vi "DVR unwrapper.vi"   [LabVIEW 2013]
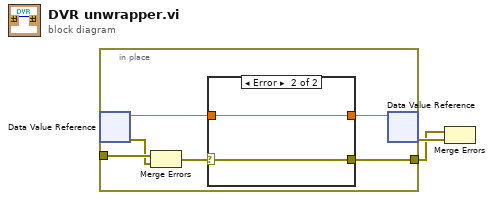
[diagram p0: block diagram]
diagram:
  n1 = in-place {
    in-place-border: _ -> [w8]
    in-place-border: [w6] -> w1
    n2 = in-place-dvr #1() -> (w3:dbl, w7:errorcluster)  [unwired: 1 in]
    n3 = Merge Errors(w8, w7) -> (w5:errorcluster)
    n4 = case shown="Error" w5 {
      selector: w5 -> [w10 w11]
      tunnel: [w10 w11] -> w6
      tunnel: [w9 w12] -> w4
      tunnel: w3 -> [w9 w12]
      frame No Error {
      }
      frame Error {
      }
    }
    n5 = in-place-dvr #1(w4) -> (w2:errorcluster)  [unwired: 1 out]
  }
  n6 = Merge Errors(w1, w2) -> ()  [unwired: 1 out]
